vi "Vision Processing.vi"(4 "error in (no error)":errorcluster, 5 "Camera Type":enum16{"206", "1011"}(ring)=enum."1011", 6 "Camera Name":string="Camera") -> ()   [LabVIEW 2011]
uses:
  Robot Global Data.vi
  <vilib>/vision/NI_Vision_Development_Module.lvlib
panel:
  in  "View":bool=TRUE
  out "Target Info":T1(array[cluster])
  in  "Area Size Limit":i32=444
  in  "Particle Count Limit":i32=8
  in  "Score Limits":T2={"Rect Coverage"=76.0, "Aspect Ratio"=70.0, "X Edge Strength"=40.0, "Y Edge Strength"=60.0}
  in  "Processing":enum32{"Color", "Intensity", "Intensity Open"}(tab)
  in  "Luminance":i32=148
  in  "Saturation":i32=55
  in  "Hue":i32(knob)=100 scale=0.0..255.0
  in  "Margins":cluster{"Hue":i32, "Sat":i32, "Lum":i32}={"Hue"=40, "Sat"=40, "Lum"=40} {"Sat" scale=0.0..40.0; "Lum" scale=0.0..40.0; "Hue" scale=0.0..40.0}
  in  "Range":cluster{"Lower value":sgl, "Upper value":sgl}={"Lower value"=150.0, "Upper value"=255.0} {"Lower value" scale=0.0..255.0; "Upper value" scale=0.0..255.0}
  in  "Range":cluster{"Lower value":sgl, "Upper value":sgl}={"Lower value"=150.0, "Upper value"=255.0} {"Lower value" scale=0.0..255.0; "Upper value" scale=0.0..255.0}
  in  "View":bool=TRUE
  out "Processed Image":T3(plugin-control)
  out "Original Image":T3(plugin-control)
  # "Instructions:\nProcessing the reflective tape that is illuminated by a ring light can be based\non color or light intensity.\nParticles within the image are scored by rectangle coverage, aspect ratio, and\nfor being hollow with a bold edge. A particle is considered a target if all scores\nare above the score limits. Particles can be annotated -- surrounded by\na rectangle and scores drawn to the left .\nTo control the number of particles being scored, use the count limit and the size\nlimit."
  # "To debug, Enable using the View button.\nFor color processing, you can click in the image to select the color for processing."
  # "Enable by clicking the View button.\nGreen scores are above the limit, orange are below. Inner/outer rect\nindicates all passed."
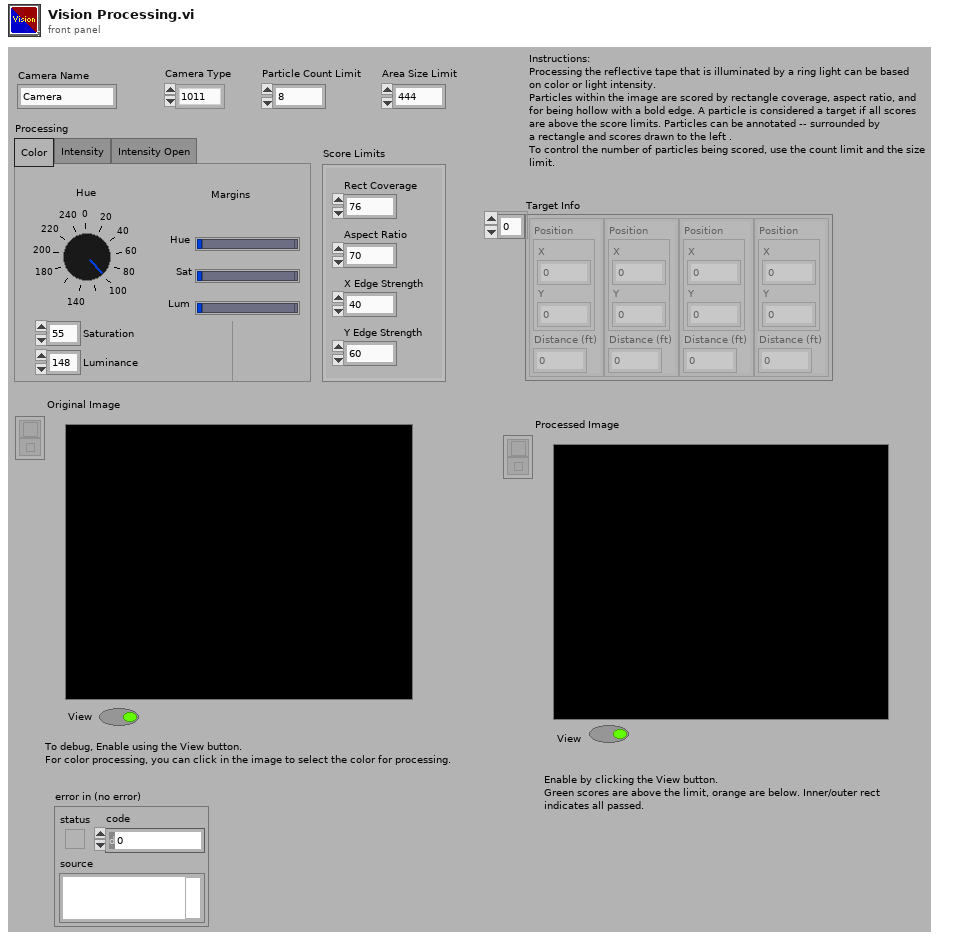
[diagram p1: front panel]
types:
  T1 = cluster{"Position":cluster{"X":dbl, "Y":dbl}, "Distance (ft)":dbl}[]
  T2 = cluster{"Rect Coverage":dbl, "Aspect Ratio":dbl, "X Edge Strength":dbl, "Y Edge Strength":dbl}
  T3 = typedef "IMAQ Image.ctl" = refnum<image>
  T4 = typedef "Image Type" = u32
  T5 = typedef "WPI_CameraDevRef.ctl" = cluster{"Camera Address":string, "CameraStatus":errorcluster, "Acquire Image Notifier":refnum<notifier>}
  T6 = enum32{"AutoM", "Close", "Dilate", "Erode", "Gradient", "Gradient out", "Gradient in", "Hit miss", "Open", "PClose", "POpen", "Thick", "Thin"}
  T7 = typedef "WPI_CameraImageSize.ctl" = enum16{"640x480", "320x240", "160x120"}
  T8 = cluster{cluster{"Left":dbl, "Top":dbl, "Right":dbl, "Bottom":dbl}, dbl[]}[]
  T9 = cluster{"Left":dbl, "Top":dbl, "Right":dbl, "Bottom":dbl}
  T10 = cluster{"Target Center (-1 to 1)":cluster{"X":dbl, "Y":dbl}, "Distance (ft)":dbl}
  T11 = cluster{"Target Center (-1 to 1)":cluster{"X":dbl, "Y":dbl}, "Distance (ft)":dbl}[]
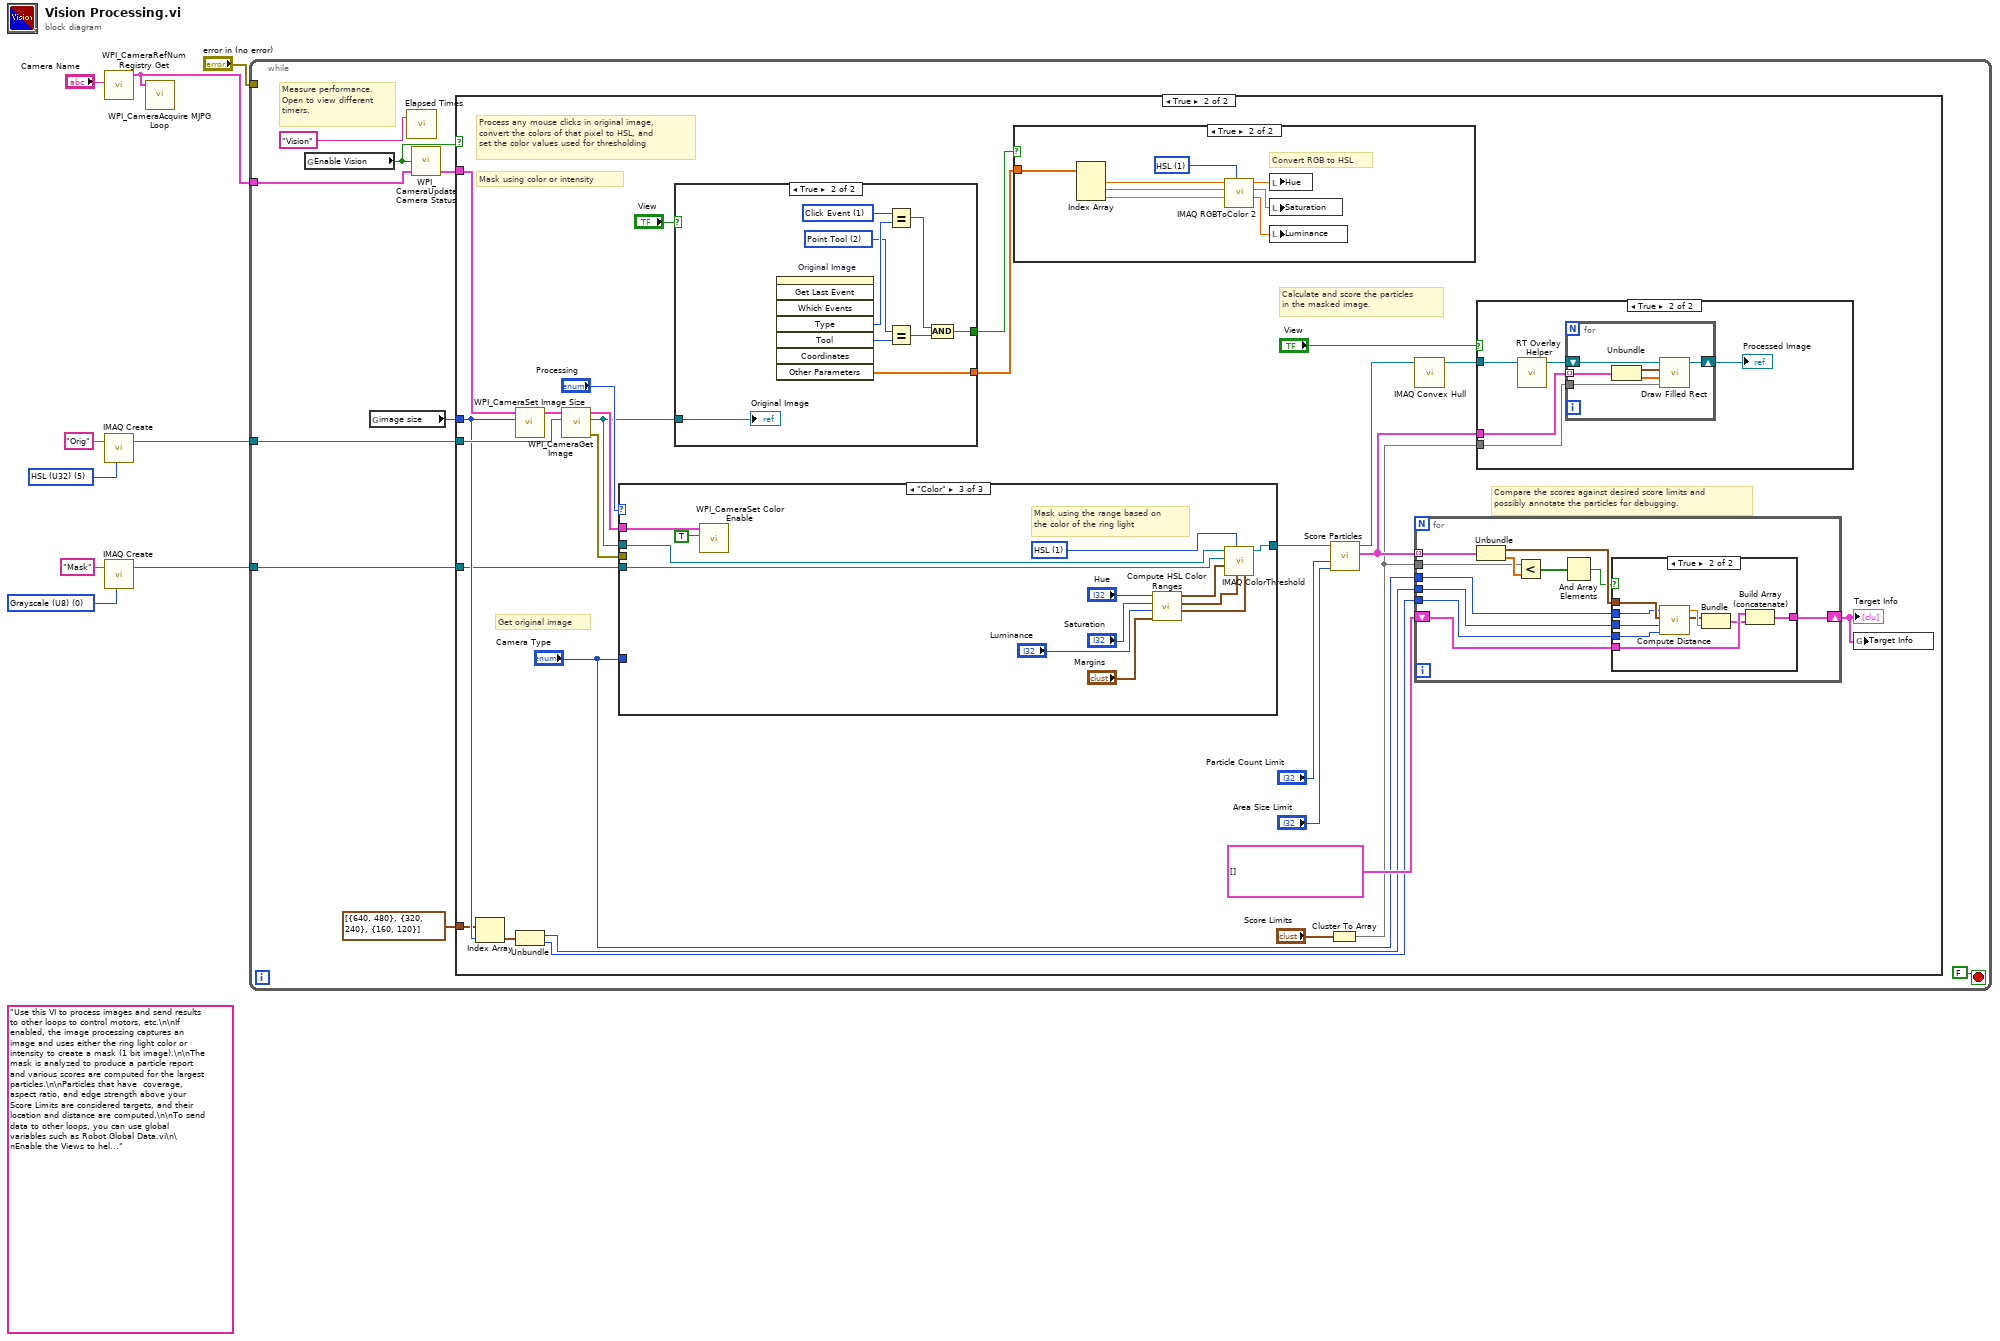
[diagram p0: block diagram]
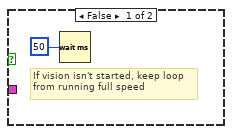
[diagram p2: hidden frame]
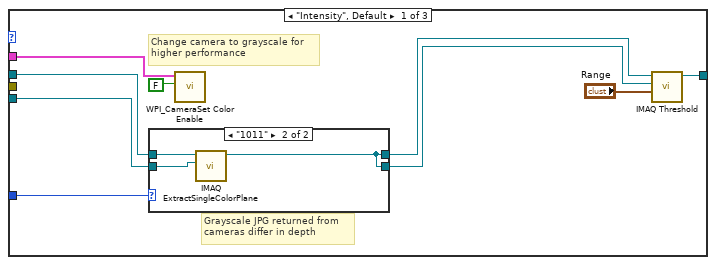
[diagram p4: hidden frame]
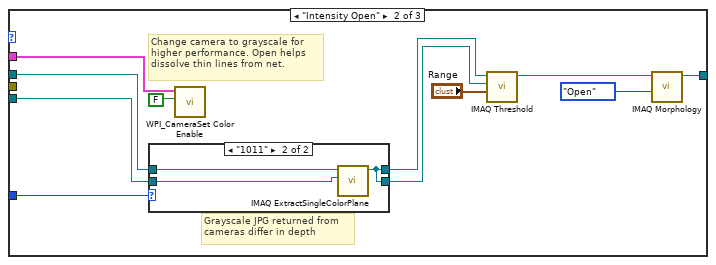
[diagram p6: hidden frame]
diagram:
  w3 = T4 0 items=["Grayscale (U8)", "Grayscale (I16)", "Grayscale (SGL)", "Complex (CSG)", "RGB (U32)", "HSL (U32)", "RGB (U64)", "Grayscale (U16)"] ("Image Type")
  (unwired) "Use this VI to process images and send results to other loops to control motors, etc.\n\nIf enabled, the image processing captures an image and uses either the ring light color or intensity to create a mask (1 bit image).\n\nThe mask is analyzed to produce a particle report and various scores are computed for the largest particles.\n\nParticles that have  coverage, aspect ratio, and edge strength above your Score Limits are considered targets, and their location and distance are computed.\n\nTo send data to other loops, you can use global variables such as Robot Global Data.vi\n\nEnable the Views to help debug color settings. Disable the View to speed up processing."
  w8 = T4 5 items=["Grayscale (U8)", "Grayscale (I16)", "Grayscale (SGL)", "Complex (CSG)", "RGB (U32)", "HSL (U32)", "RGB (U64)", "Grayscale (U16)"] ("Image Type")
  n1 = call <vilib>:"WPI_CameraRefNum Registry Get.vi"("refnum name"="Camera Name") -> ("CameraDevRef"=w5:T5)  [unwired: 9 in, 1 out]
  n2 = call "IMAQ Create"("Image Name"="Orig", "Image Type"=w8) -> ("New Image"=w7:T3)  [unwired: 2 in, 2 out]
  n3 = call "IMAQ Create"("Image Name"="Mask", "Image Type"=w3) -> ("New Image"=w1:T3)  [unwired: 2 in, 2 out]
  n4 = call <vilib>:"WPI_CameraAcquire MJPG Loop.vi"("CameraDevRef"=w5) -> ()  [unwired: 11 in]
  n5 = while {
    tunnel: w7 -> [w17]
    tunnel: w5 -> [w16]
    tunnel: "error in (no error)" -> [_]
    tunnel: w1 -> [w11]
    stop <- FALSE stop-if-true
    # "Measure performance.\nOpen to view different\ntimers."
    n6 = global read "Robot Global Data.vi" "Enable Vision"() -> (w14:bool)
    n7 = global read "Robot Global Data.vi" "image size"() -> (w12:T7)
    n8 = call "Elapsed Times.vi"("Call Name"="Vision") -> ()  [unwired: 2 in, 1 out]
    n9 = call <vilib>:"WPI_CameraUpdate Camera Status.vi"("CameraDevRef In"=w16, "Enable Vision"=w14) -> ("CameraDevRef Out"=w15:T5)  [unwired: 3 in]
    n10 = case shown="True" w14 {
      tunnel: w17 -> [_ w39]
      tunnel: w15 -> [_ w34]
      tunnel: w12 -> [_ w30]
      tunnel: w11 -> [_ w25]
      tunnel: cluster{i32, i32}[] [{640, 480}, {320, 240}, {160, 120}] -> [_ w29]
      frame False {
        # "If vision isn't started, keep loop\nfrom running full speed"
        n11 = Wait (ms)(milliseconds to wait=u32 50) -> ()  [unwired: 1 out]
      }
      frame True {
        # "Compare the scores against desired score limits and\npossibly annotate the particles for debugging."
        # "Process any mouse clicks in original image,\nconvert the colors of that pixel to HSL, and\nset the color values used for thresholding"
        # "Calculate and score the particles\nin the masked image."
        # "Mask using color or intensity"
        # "Get original image"
        n12 = Index Array(array=w29, index=w30) -> (element=w26:cluster{i32, i32})
        n13 = call <vilib>:"WPI_CameraSet Image Size.vi"("Image Size"=w30, "CameraDevRef"=w34) -> ("CameraDevRef Out"=w35:T5)  [unwired: 8 in, 1 out]
        n14 = Unbundle(w26) -> (w28:i32, w27:i32)
        n15 = call <vilib>:"WPI_CameraGet Image.vi"("Image"=w39, "CameraDevRef"=w35) -> ("error out"=w37:errorcluster, "Image Out"=w24:T3, "CameraDevRef Out"=w38:T5)  [unwired: 7 in]
        n16 = case shown="\"Color\"" "Processing" {
          tunnel: w24 -> [w60 w72 w98]
          tunnel: [w63 w77 w97] -> w22
          tunnel: w38 -> [w61 w75 w88]
          tunnel: w37 -> [_ _ _]
          tunnel: w25 -> [w59 w73 w86]
          tunnel: "Camera Type" -> [w58 w74 _]
          frame "Intensity", Default {
            # "Grayscale JPG returned from\ncameras differ in depth"
            # "Change camera to grayscale for\nhigher performance"
            n17 = case shown="\"1011\"" w58 {
              tunnel: w60 -> [w66 w69]
              tunnel: w59 -> [w65 w68]
              tunnel: [w66 w67] -> w57
              tunnel: [w65 w67] -> w56
              frame "206", Default {
              }
              frame "1011" {
                n18 = call "IMAQ ExtractSingleColorPlane"("Image Dst"=w68, "Image Src"=w69) -> ("Image Dst Out"=w67:T3)  [unwired: 8 in, 1 out]
              }
            }
            n19 = call <vilib>:"WPI_CameraSet Color Enable.vi"("Color Enabled"=FALSE, "CameraDevRef"=w61) -> ()  [unwired: 8 in, 2 out]
            n20 = call "IMAQ Threshold"("Range"="Range", "Image Dst"=w56, "Image Src"=w57) -> ("Image Dst Out"=w63:T3)  [unwired: 3 in, 5 out]
          }
          frame "Intensity Open" {
            # "Grayscale JPG returned from\ncameras differ in depth"
            # "Change camera to grayscale for\nhigher performance. Open helps\ndissolve thin lines from net."
            n21 = case shown="\"1011\"" w74 {
              tunnel: w72 -> [w82 w85]
              tunnel: w73 -> [w81 w84]
              tunnel: [w82 w83] -> w71
              tunnel: [w81 w83] -> w70
              frame "206", Default {
              }
              frame "1011" {
                n22 = call "IMAQ ExtractSingleColorPlane"("Image Dst"=w84, "Image Src"=w85) -> ("Image Dst Out"=w83:T3)  [unwired: 8 in, 1 out]
              }
            }
            n23 = call <vilib>:"WPI_CameraSet Color Enable.vi"("Color Enabled"=FALSE, "CameraDevRef"=w75) -> ()  [unwired: 8 in, 2 out]
            n24 = call "IMAQ Threshold"("Range"="Range", "Image Dst"=w70, "Image Src"=w71) -> ("Image Dst Out"=w78:T3)  [unwired: 3 in, 5 out]
            n25 = call "IMAQ Morphology"("Operation"=T6."Open", "Image Src"=w78) -> ("Image Dst Out"=w77:T3)  [unwired: 8 in, 1 out]
          }
          frame "Color" {
            w96 = u16 1 items=["RGB", "HSL", "HSV", "HSI"] ("Color Mode")
            # "Mask using the range based on\nthe color of the ring light"
            n26 = call <vilib>:"WPI_CameraSet Color Enable.vi"("Color Enabled"=TRUE, "CameraDevRef"=w88) -> ()  [unwired: 8 in, 2 out]
            n27 = call "Compute HSL Color Ranges.vi"("Margins"="Margins", "Luminance"="Luminance", "Saturation"="Saturation", "Hue"="Hue") -> ("Lum Range"=w93:cluster{i32, i32}, "Sat Range"=w94:cluster{i32, i32}, "Hue Range"=w95:cluster{i32, i32})  [unwired: 5 in]
            n28 = call "IMAQ ColorThreshold"("Blue or Luma or Val or Inten Range"=w93, "Green or Sat Range"=w94, "Color Mode"=w96, "Red or Hue Range"=w95, "Image Dst"=w86, "Image Src"=w98) -> ("Image Dst Out"=w97:T3)  [unwired: 4 in, 1 out]
          }
        }
        n29 = case shown="True" "View" {
          tunnel: w24 -> [_ w118]
          tunnel: [_ w113] -> w32
          tunnel: [_ w110] -> w31
          frame False {
          }
          frame True {
            w111 = 2 items=["None", "Selection Tool", "Point Tool", "Line Tool", "Rectangle Tool", "Oval Tool", "Polygon Tool", "ClosedFreehandTool", "Annulus Tool", "Rotated Rectangle Tool", "Zoom Tool", "Pan Tool", "Polyline Tool", "Freehand Tool"] ("Tool")
            w112 = 1 items=["No Event"=0, "Click Event"=1, "Draw Event"=2, "Size Event"=4, "Scroll Event"=5, "Double Click Event"=8] ("Type")
            n30 = invoke on="Original Image" class="ImageControl" method="Get Last Event"() -> ("Type"=w114:i32, "Tool"=w117:i32, "Other Parameters"=w110:sgl[])  [unwired: 8 in, 5 out]
            n31 = Equal?(x=w112, y=w114) -> (x = y?=w115:bool)
            n32 = Equal?(x=w111, y=w117) -> (x = y?=w116:bool)
            n33 = And(x=w115, y=w116) -> (x .and. y?=w113:bool)
            "Original Image" <- w118
          }
        }
        n34 = case shown="True" w32 {
          tunnel: w31 -> [_ w55]
          frame False {
          }
          frame True {
            w54 = u16 1 items=["RGB", "HSL", "HSV", "HSI", "CIE L*a*b*", "CIE XYZ"] ("Color Mode")
            # "Convert RGB to HSL"
            n35 = Index Array(array=w55) -> (element #1=w53:sgl, element #2=w51:sgl, element #3=w49:sgl)  [unwired: 3 in]
            n36 = call "IMAQ RGBToColor 2"("Color Mode"=w54, "Blue value"=w49, "Green value"=w51, "Red value"=w53) -> ("Blue or Luma or Val or Inten or Z or b*value"=w48:dbl, "Green or Sat or Y or a* value"=w50:dbl, "Red or Hue or X or L* value"=w52:dbl)  [unwired: 4 in, 1 out]
            n37 = local write "Hue"(w52) -> ()
            n38 = local write "Saturation"(w50) -> ()
            n39 = local write "Luminance"(w48) -> ()
          }
        }
        n40 = Cluster To Array(cluster="Score Limits") -> (array=w42:dbl[])
        n41 = call "Score Particles.vi"("Area Size Limit"="Area Size Limit", "Particle Count Limit"="Particle Count Limit", "Image Refnum in"=w22) -> ("Scored Particle Info"=w44:T8, "Image Refnum out"=w20:T3)  [unwired: 7 in]
        n42 = call "IMAQ Convex Hull"("Image Src"=w20) -> ("Image Dst Out"=w21:T3)  [unwired: 9 in, 1 out]
        n43 = for {
          shift-right: [w128] -> w36
          shift-left: T1 [] -> [w129]
          tunnel: w28 -> [w127]
          tunnel: w44 -> [w125] mode=indexing
          tunnel: w42 -> [w120]
          tunnel: "Camera Type" -> [w124]
          tunnel: w27 -> [w119]
          n44 = Unbundle(w125) -> (w126:T9, w121:dbl[])
          n45 = Less?(x=w120, y=w121) -> (x < y?=w123:bool[])
          n46 = And Array Elements(Boolean array=w123) -> (logical AND=w122:bool)
          n47 = case shown="True" w122 {
            tunnel: w129 -> [w130 w139]
            tunnel: [w130 w138] -> w128
            tunnel: w126 -> [_ w134]
            tunnel: w127 -> [_ w136]
            tunnel: w124 -> [_ w133]
            tunnel: w119 -> [_ w132]
            frame False {
            }
            frame True {
              n48 = call "Compute Distance.vi"("Y Image Resolution"=w132, "X Image Resolution"=w136, "Bounding Box"=w134, "Camera Type"=w133) -> ("Target Center (-1 to 1)"=w131:cluster{"X":dbl, "Y":dbl}, "Distance (ft)"=w135:dbl)  [unwired: 6 in]
              n49 = Bundle("Target Center (-1 to 1)"=w131, "Distance (ft)"=w135) -> (w137:T10)  [unwired: 1 in]
              n50 = Build Array (concatenate)(w139, w137) -> (w138:T11)
            }
          }
        }
        "Target Info" <- w36
        n51 = case shown="True" "View" {
          tunnel: w21 -> [_ w100]
          tunnel: w44 -> [_ w102]
          tunnel: w42 -> [_ w101]
          frame False {
          }
          frame True {
            n52 = call "RT Overlay Helper.vi"("Refnum in"=w100) -> ("Refnum out"=w103:T3)  [unwired: 10 in]
            n53 = for {
              shift-right: [w108] -> w99
              shift-left: w103 -> [w109]
              tunnel: w102 -> [w105] mode=indexing
              tunnel: w101 -> [w104]
              n54 = Unbundle(w105) -> (w106:T9, w107:dbl[])
              n55 = call "Draw Filled Rect.vi"("Limits"=w104, "Scores"=w107, "Bounding Box"=w106, "image in"=w109) -> ("image out"=w108:T3)  [unwired: 7 in]
            }
            "Processed Image" <- w99
          }
        }
        n56 = global write "Robot Global Data.vi" "Target Info"(w36) -> ()
      }
    }
  }
